vi "Create HTML For String Color.vi"(8 "error in":errorcluster, 11 "GObject in":refnum<vi>) -> (0 "error out":errorcluster, 1 "Text Color":string, 2 "Background Color":string, 3 "Style For Color":string, 4 "Size":string, 5 "Border":string, 6 "Weight":string, 7 "Justify":string)   [LabVIEW 2015, in "Front Panel Publisher.lvlib" / "String.lvclass"]
uses:
  String.lvclass
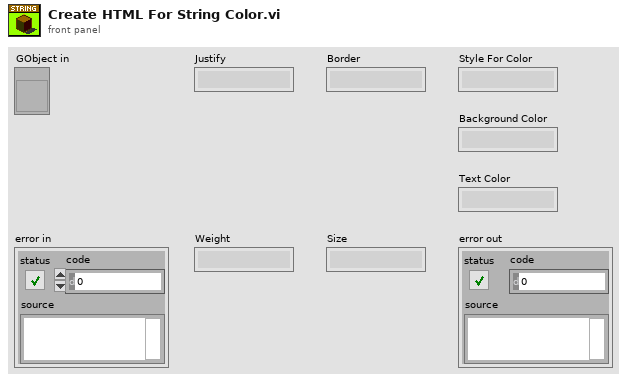
[diagram p1: front panel]
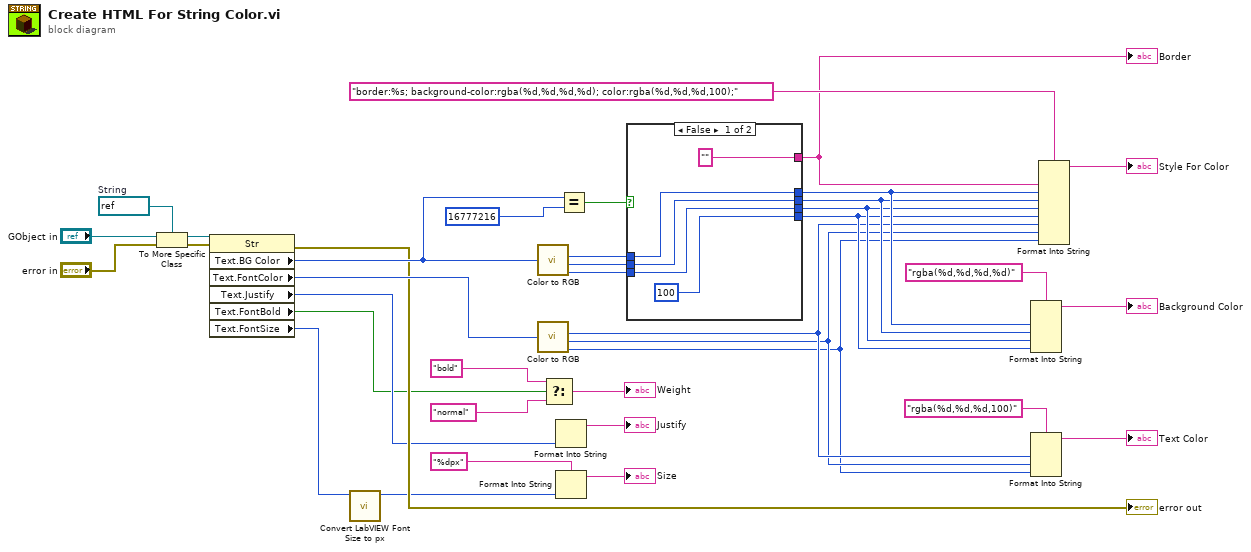
[diagram p0: block diagram]
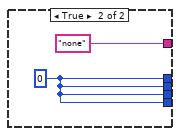
[diagram p2: hidden frame]
diagram:
  w36 = refnum<vi> refnum  # String
  n1 = To More Specific Class(target class=w36, reference="GObject in", error in="error in") -> (specific class reference=w35:refnum<vi>, error out=w34:errorcluster)
  n2 = property class="Str"(reference=w35, error in=w34) -> (error out=→"error out":errorcluster, "Text.BG Color"=w31:u32, "Text.FontColor"=w26:u32, "Text.Justify"=w10:enum16{"Left", "Center", "Right"}, "Text.FontBold"=w6:bool, "Text.FontSize"=w2:u32)  [unwired: 1 out]
  n3 = call "Convert LabVIEW Font Size to px.vi"("LabVIEW Font Size"=w2) -> ("px Font Size"=w1:i32)  [unwired: 10 in]
  n4 = call <vilib>:"Color to RGB.vi"("Color"=w31) -> ("R"=w30:u8, "G"=w29:u8, "B"=w28:u8)  [unwired: 1 out]
  n5 = call <vilib>:"Color to RGB.vi"("Color"=w26) -> ("R"=w17:u8, "G"=w16:u8, "B"=w15:u8)  [unwired: 1 out]
  n6 = Select(t="bold", s=w6, f="normal") -> (s? t:f=→"Weight":string)
  n7 = Format Into String(w10) -> (resulting string=→"Justify":string)  [unwired: 3 in, 1 out]
  n8 = Format Into String(format string="%dpx", w1) -> (resulting string=→"Size":string)  [unwired: 2 in, 1 out]
  n9 = Equal?(x=w31, y=u32 16777216) -> (x = y?=w32:bool)
  n10 = case shown="False" w32 {
    tunnel: [w42 w44] -> w21
    tunnel: w30 -> [w42 _]
    tunnel: [w41 w44] -> w20
    tunnel: w29 -> [w41 _]
    tunnel: [w40 w44] -> w19
    tunnel: w28 -> [w40 _]
    tunnel: [u8 100 ("B") w44] -> w18
    tunnel: ["" "none"] -> w27
    frame False {
    }
    frame True {
      w44 = u8 0 ("R")
    }
  }
  "Border" <- w27
  n11 = Format Into String(format string="rgba(%d,%d,%d,%d)", w21, w20, w19, w18) -> (resulting string=→"Background Color":string)  [unwired: 2 in, 1 out]
  n12 = Format Into String(format string="rgba(%d,%d,%d,100)", w17, w16, w15) -> (resulting string=→"Text Color":string)  [unwired: 2 in, 1 out]
  n13 = Format Into String(format string="border:%s; background-color:rgba(%d,%d,%d,%d); color:rgba(%d,%d,%d,100);", w27, w21, w20, w19, w18, w17, w16, w15) -> (resulting string=→"Style For Color":string)  [unwired: 2 in, 1 out]
